vi "Periodic Tasks.vi"(8 "error in":errorcluster) -> ()   [LabVIEW 2019]
doc: "This VI runs in parallel to other tasks. It can contain as many user-defined periodic loops as you need. These can carry out PID or other sorts of timed response."
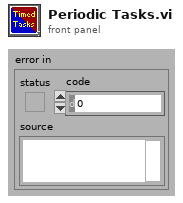
[diagram p1: front panel]
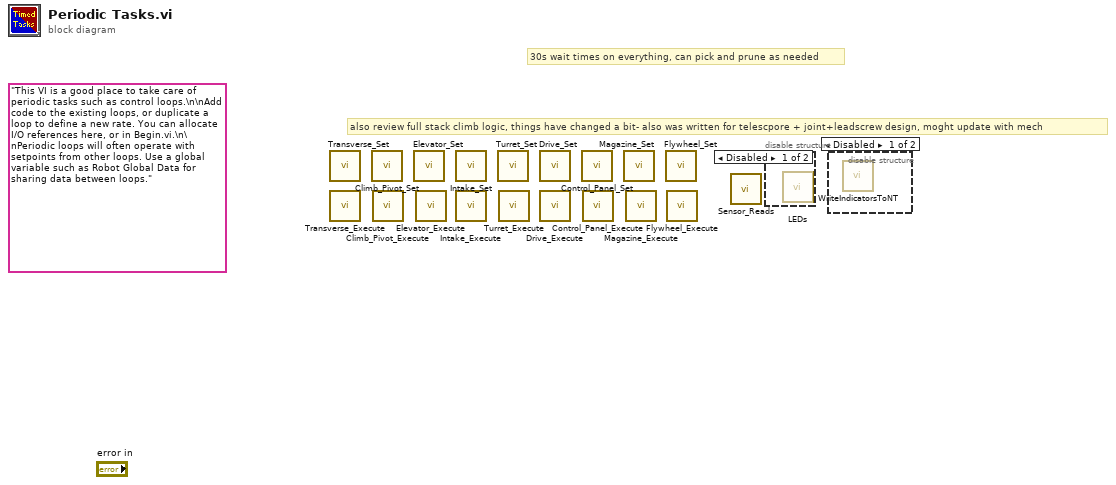
[diagram p0: block diagram]
diagram:
  (unwired) "This VI is a good place to take care of periodic tasks such as control loops.\n\nAdd code to the existing loops, or duplicate a loop to define a new rate. You can allocate I/O references here, or in Begin.vi.\n\nPeriodic loops will often operate with setpoints from other loops. Use a global variable such as Robot Global Data for sharing data between loops."
  # "30s wait times on everything, can pick and prune as needed"
  # "also review full stack climb logic, things have changed a bit- also was written for telescpore + joint+leadscrew design, moght update with mech"
  n1 = call "Transverse_Set.vi"() -> ()  [unwired: 12 in]
  n2 = call "Transverse_Execute.vi"() -> ()  [unwired: 12 in]
  n3 = call "Climb_Pivot_Set.vi"() -> ()  [unwired: 12 in]
  n4 = call "Climb_Pivot_Execute.vi"() -> ()  [unwired: 12 in]
  n5 = call "Elevator_Set.vi"() -> ()  [unwired: 12 in]
  n6 = call "Elevator_Execute.vi"() -> ()  [unwired: 12 in]
  n7 = call "Intake_Set.vi"() -> ()  [unwired: 12 in]
  n8 = call "Intake_Execute.vi"() -> ()  [unwired: 12 in]
  n9 = call "Turret_Set.vi"() -> ()  [unwired: 12 in]
  n10 = call "Turret_Execute.vi"() -> ()  [unwired: 12 in]
  n11 = call "Drive_Set.vi"() -> ()  [unwired: 12 in]
  n12 = call "Drive_Execute.vi"() -> ()  [unwired: 12 in]
  n13 = call "Control_Panel_Set.vi"() -> ()  [unwired: 12 in]
  n14 = call "Control_Panel_Execute.vi"() -> ()  [unwired: 12 in]
  n15 = call "Magazine_Set.vi"() -> ()  [unwired: 12 in]
  n16 = call "Magazine_Execute.vi"() -> ()  [unwired: 12 in]
  n17 = call "Flywheel_Set.vi"() -> ()  [unwired: 12 in]
  n18 = call "Flywheel_Execute.vi"() -> ()  [unwired: 12 in]
  n19 = call "Sensor_Reads.vi"() -> ()  [unwired: 12 in]
  n20 = disable-structure shown="Disabled" {
    frame Disabled {
      n21 = call "LEDs.vi"() -> ()  [unwired: 12 in]
    }
    frame Enabled {
    }
  }
  n22 = disable-structure shown="Disabled" {
    frame Disabled {
      n23 = call "WriteIndicatorsToNT.vi"() -> ()  [unwired: 12 in]
    }
    frame Enabled {
    }
  }
